vi "Process Data Buffer, Mode 0.vi"(0 "DATA_Buffer excluding '#' [1...N]":string, 1 "P constants":T1[](array[typedef])) -> (2 "Pressures":sgl[](array[numeric]), 3 "Statuses":u8[](array[numeric]), 4 "dt_warn":u8)   [LabVIEW 2020]
uses:
  Ctls/Pressure sensor constants.ctl
panel:
  # "0: valid data\n1: cmd mode\n2: stale data\n3: diag mode"
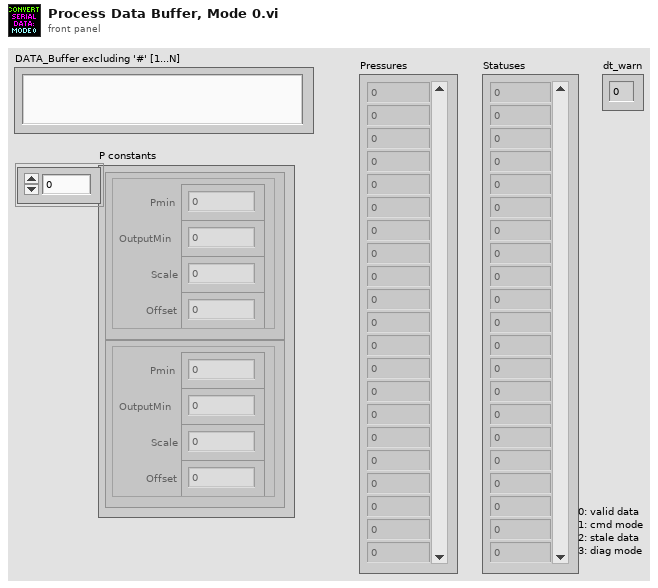
[diagram p1: front panel]
types:
  T1 = typedef "Pressure sensor constants.ctl" = cluster{"Pmin":sgl, "OutputMin":sgl, "Scale":sgl, "Offset":sgl}
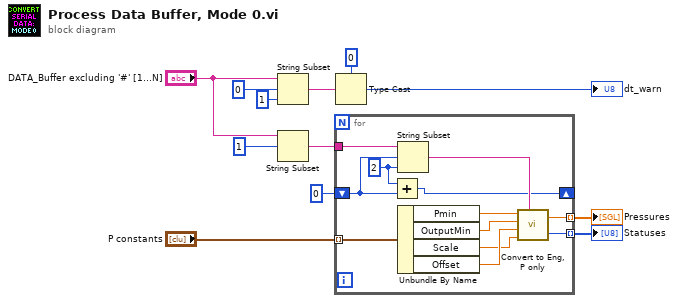
[diagram p0: block diagram]
diagram:
  n1 = String Subset(string="DATA_Buffer excluding '#' [1...N]", offset (0)=0, length (rest)=1 ("length (rest)")) -> (substring=w10:string)
  n2 = String Subset(string="DATA_Buffer excluding '#' [1...N]", offset (0)=1) -> (substring=w5:string)  [unwired: 1 in]
  n3 = for {
    tunnel: w5 -> [w22]
    tunnel: [w24] -> w2 mode=indexing
    tunnel: [w23] -> w1 mode=indexing
    shift-right: [w19] -> _
    shift-left: 0 ("offset (0)") -> [w18]
    tunnel: "P constants" -> [w17] mode=indexing
    w20 = 2 ("length (rest)")
    n4 = Add(x=w20, y=w18) -> (x+y=w19:i32)
    n5 = String Subset(string=w22, offset (0)=w18, length (rest)=w20) -> (substring=w21:string)
    n6 = Unbundle By Name(w17) -> ("Pmin"=w16:sgl, "OutputMin"=w15:sgl, "Scale"=w13:sgl, "Offset"=w14:sgl)
    n7 = call "Convert to Eng, P only.vi"("Pmin (Pa)"=w16, "OutputMin (counts)"=w15, "Poffset (Pa)"=w14, "(Pmax - Pmin) / (OutputMax - OutputMin) (Pa/count)"=w13, "P word"=w21) -> ("P (Pa)"=w24:sgl, "Status bits"=w23:u8)
  }
  "Pressures" <- w2
  "Statuses" <- w1
  n8 = Type Cast(type=u8 0, x=w10) -> (*(type *) &x=→"dt_warn":u8)
